vi "Init.vi"(8 "error in (no error)":errorcluster, 11 "ImageHandler in":refnum<class "ImageHandler.lvclass">) -> (0 "error out":errorcluster, 3 "ImageHandler out":refnum<class "ImageHandler.lvclass">)   [LabVIEW 2022 SP3, in "ImageHandler.lvlib" / "ImageHandler.lvclass"]
uses:
  ImageHandler.lvclass
  C:/Program Files/National Instruments/LabVIEW 2022/vi.lib/ActorFramework/Actor/Actor.lvclass
  <vilib>/ActorFramework/Actor/Actor.lvclass/Actor.ctl
  ImageHandler - Controller -- Interface/ImageHandler - Controller -- Interface Messages/Connection Status Msg/Connection Status Msg.lvclass/Connection Status Msg.ctl
  <vilib>/ActorFramework/Message Enqueuer/Message Enqueuer.lvclass/Message Enqueuer.ctl
  <vilib>/ActorFramework/Message Enqueuer/Enqueue.vi
  ImageHandler - Controller -- Interface/ImageHandler - Controller -- Interface Messages/Connection Status Msg/Connection Status Msg.lvclass
  C:/Program Files/National Instruments/LabVIEW 2022/vi.lib/ActorFramework/Message/Message.lvclass
  <vilib>/ActorFramework/Message Priority Queue/Priority Enqueue.vi
  ImageHandler.lvclass/ImageHandler.ctl
  <vilib>/ActorFramework/Actor/Actor.lvclass
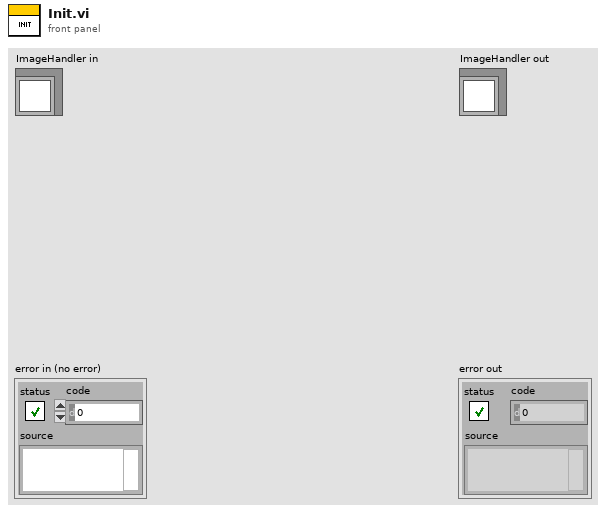
[diagram p1: front panel]
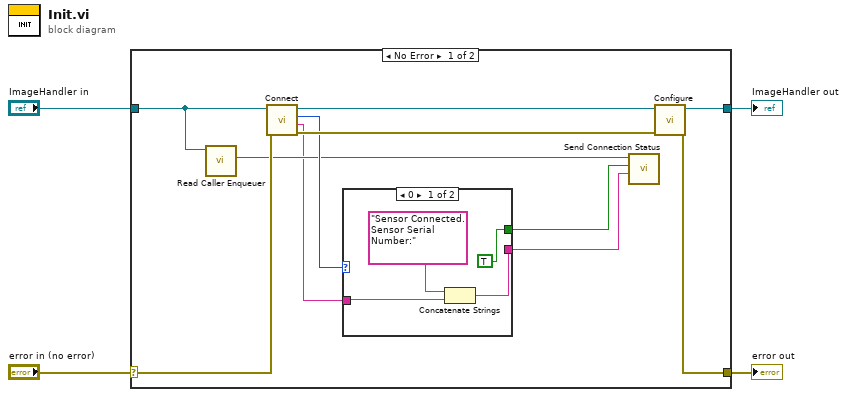
[diagram p0: block diagram]
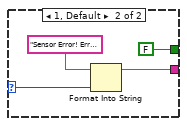
[diagram p2: hidden frame]
diagram:
  n1 = case shown="No Error" "error in (no error)" {
    selector: "error in (no error)" -> [w15 w25]
    tunnel: [w5 w25] -> w3
    tunnel: [w12 w24] -> w1
    tunnel: "ImageHandler in" -> [w10 w24]
    frame No Error {
      n2 = call <vilib>:"Read Caller Enqueuer.vi"("Actor"=w10) -> ("Caller Enqueuer"=w9:refnum<class "Message Enqueuer.lvclass">)  [unwired: 10 in]
      n3 = call "Connect.vi"("error in (no error)"=w15, "ImageHandler in"=w10) -> ("error out"=w14:errorcluster, "Serial Number"=w7:string, "Sensor Status"=w11:i32, "ImageHandler out"=w13:refnum<class "ImageHandler.lvclass">)  [unwired: 6 in]
      n4 = case shown="0" w11 {
        selector: w11 -> [_ w22]
        tunnel: [TRUE FALSE] -> w8
        tunnel: w7 -> [w17 _]
        tunnel: [w16 w20] -> w6
        frame 0 {
          n5 = Concatenate Strings("Sensor Connected. Sensor Serial Number:", w17) -> (w16:string)
        }
        frame 1, Default {
          n6 = Format Into String(initial string="Sensor Error! Error Code:", w22) -> (resulting string=w20:string)  [unwired: 2 in, 1 out]
        }
      }
      n7 = call "Send Connection Status.vi"("Remarks"=w6, "Status"=w8, "Message Enqueuer"=w9) -> ()  [unwired: 7 in, 2 out]
      n8 = call "Configure.vi"("error in (no error)"=w14, "ImageHandler in"=w13) -> ("error out"=w5:errorcluster, "ImageHandler out"=w12:refnum<class "ImageHandler.lvclass">)  [unwired: 8 in]
    }
    frame Error {
    }
  }
  "error out" <- w3
  "ImageHandler out" <- w1
